vi "DSF.Engine.Plugin.Tx (old).vi"(8 "error in (no error)":errorcluster, 10 "Transfer Group in":refnum<class "DSF.Engine.Transfer Group.lvclass">, 11 "Plugin in":refnum<class "DSF.Engine.Plugin.lvclass">) -> (0 "error out":errorcluster, 2 "Transfer Group out":refnum<class "DSF.Engine.Transfer Group.lvclass">, 3 "Plugin out":refnum<class "DSF.Engine.Plugin.lvclass">)   [LabVIEW 2017, in "DSF.Engine.lvlib" / "DSF.Engine.Plugin.lvclass"]
uses:
  DSF.Engine.Plugin.lvclass
  Transfer/DSF.Engine.Transfer Group.lvclass
  DSF.Engine.Plugin.lvclass/DSF.Engine.Plugin.ctl
  Transceiver/DSF.Engine.Transceiver.lvclass
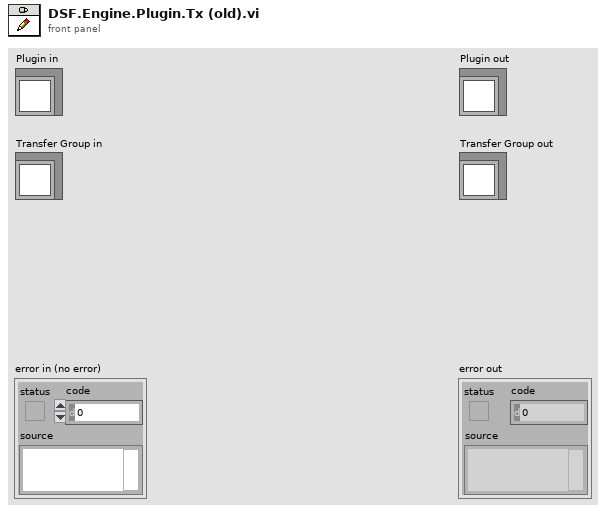
[diagram p1: front panel]
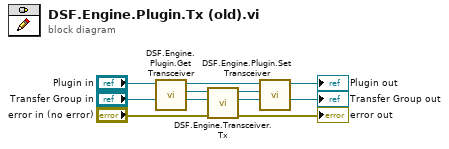
[diagram p0: block diagram]
diagram:
  n1 = call "DSF.Engine.Plugin.Get Transceiver.vi"("Plugin in"="Plugin in") -> ("Transceiver"=w9:refnum<class "DSF.Engine.Transceiver.lvclass">, "Plugin out"=w7:refnum<class "DSF.Engine.Plugin.lvclass">)  [unwired: 9 in]
  n2 = call-dynamic "DSF.Engine.Transceiver.Tx.vi"("error in (no error)"="error in (no error)", "Transfer Group in"="Transfer Group in", "Transceiver in"=w9) -> ("error out"=→"error out":errorcluster, "Transfer Group out"=→"Transfer Group out":refnum<class "DSF.Engine.Transfer Group.lvclass">, "Transceiver out"=w8:refnum<class "DSF.Engine.Transceiver.lvclass">)  [unwired: 6 in]
  n3 = call "DSF.Engine.Plugin.Set Transceiver.vi"("Transceiver"=w8, "Plugin in"=w7) -> ("Plugin out"=→"Plugin out":refnum<class "DSF.Engine.Plugin.lvclass">)  [unwired: 9 in]
